vi "all_things_stimulus.vi"(1 "input cluster":T1) -> (0 "output cluster":T2)   [LabVIEW 2010]
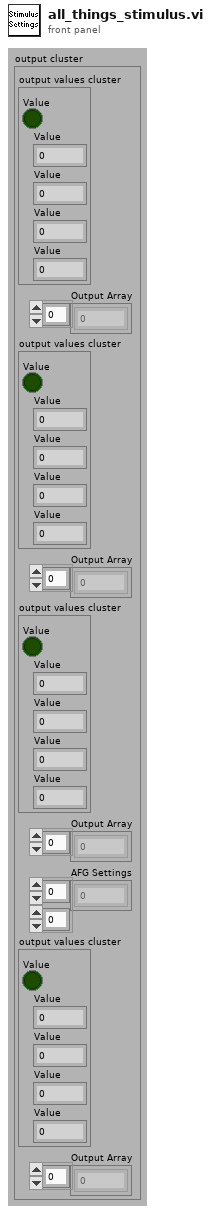
[diagram p1: front panel]
types:
  T1 = cluster{"AFG Settings":dbl[][], "tap timing array":dbl[], "puff timing array":dbl[], "custom timing array":dbl[], "custom 2 timing array":dbl[], cluster{cluster{"Tap":refnum<vi>, "Tap Delay":refnum<vi>, "Tap Interval":refnum<vi>, "Tap Number":refnum<vi>, "Tap Stimulus Method":refnum<vi>}, cluster{"Puff":refnum<vi>, "Puff Delay":refnum<vi>, "Puff Interval":refnum<vi>, "Puff Number":refnum<vi>, "Puff Stimulus Method":refnum<vi>}, cluster{"Custom 1":refnum<vi>, "Custom 1 Delay":refnum<vi>, "Custom 1 Interval":refnum<vi>, "Custom 1 Number":refnum<vi>, "Custom 1 Stimulus Method":refnum<vi>}, cluster{"Custom 2":refnum<vi>, "Custom 2 Delay":refnum<vi>, "Custom 2 Interval":refnum<vi>, "Custom 2 Number":refnum<vi>, "Custom 2 Stimulus Method":refnum<vi>}}, cluster{"Path":refnum<vi>, "Prefix":refnum<vi>, "Type of object to track":refnum<vi>, "Object Contrast (%)":refnum<vi>, "Fill Hysteresis (%)":refnum<vi>, "Maximum Object Size (pixels)":refnum<vi>, "Minimum Object Size (pixels)":refnum<vi>, "Object Size hysteresis (%)":refnum<vi>, "Image Binning":refnum<vi>, "Contour?":refnum<vi>, "Skeletonize?":refnum<vi>, "Frames of Adaptation":refnum<vi>, "Adaptation Rate":refnum<vi>, "Object Border":refnum<vi>, "Image Bit Depth":refnum<vi>, "Bit Depth from Camera?":refnum<vi>, "AFG resource name":refnum<vi>, "IMAQ Camera Interface Name":refnum<vi>, "Device auto-start delay (s)":refnum<vi>, "Number of Image Adaptation Bands":refnum<vi>, "Experiment Duration (s)":refnum<vi>, "Tap":refnum<vi>, "Tap Delay":refnum<vi>, "Tap Interval":refnum<vi>, "Tap Number":refnum<vi>, "Tap Stimulus Method":refnum<vi>, "Advanced Tap Settings":refnum<vi>, "Puff":refnum<vi>, "Puff Delay":refnum<vi>, "Puff Interval":refnum<vi>, "Puff Number":refnum<vi>, "Puff Stimulus Method":refnum<vi>, "Advanced Puff Settings":refnum<vi>, "Custom 1":refnum<vi>, "Custom 1 Delay":refnum<vi>, "Custom 1 Interval":refnum<vi>, "Custom 1 Number":refnum<vi>, "Custom 1 Stimulus Method":refnum<vi>, "Advanced Custom 1 Settings":refnum<vi>, "puff fraction of time between is active":refnum<vi>, "time between puff onset":refnum<vi>, "tap fraction of time between is active":refnum<vi>, "time between tap onset":refnum<vi>, "Tap Train Number":refnum<vi>, "custom 1 fraction of time between is active":refnum<vi>, "time between custom 1 onset":refnum<vi>, "Custom 2":refnum<vi>, "Custom 2 Delay":refnum<vi>, "Custom 2 Interval":refnum<vi>, "Custom 2 Number":refnum<vi>, "Custom 2 Stimulus Method":refnum<vi>, "Advanced Custom 2 Settings":refnum<vi>, "custom 2 fraction of time between is active":refnum<vi>, "time between custom 2 onset":refnum<vi>, "Save":refnum<vi>, "Load":refnum<vi>, "Raw Image Save Interval (s)":refnum<vi>, "Turn on output aggregation?":refnum<vi>, "Turn on Background division algorithm":refnum<vi>, "Turn on external triggering of camera":refnum<vi>}, "output values cluster":cluster{"Value":bool, "Value":dbl, "Value":dbl, "Value":dbl, "Value":u16}, "output values cluster":cluster{"Value":bool, "Value":dbl, "Value":dbl, "Value":dbl, "Value":u16}, "output values cluster":cluster{"Value":bool, "Value":dbl, "Value":dbl, "Value":dbl, "Value":u16}, "output values cluster":cluster{"Value":bool, "Value":dbl, "Value":dbl, "Value":dbl, "Value":u16}}
  T2 = cluster{"output values cluster":cluster{"Value":bool, "Value":dbl, "Value":dbl, "Value":dbl, "Value":u16}, "Output Array":dbl[], "output values cluster":cluster{"Value":bool, "Value":dbl, "Value":dbl, "Value":dbl, "Value":u16}, "Output Array":dbl[], "output values cluster":cluster{"Value":bool, "Value":dbl, "Value":dbl, "Value":dbl, "Value":u16}, "Output Array":dbl[], "AFG Settings":dbl[][], "output values cluster":cluster{"Value":bool, "Value":dbl, "Value":dbl, "Value":dbl, "Value":u16}, "Output Array":dbl[]}
  T3 = cluster{cluster{"Tap":refnum<vi>, "Tap Delay":refnum<vi>, "Tap Interval":refnum<vi>, "Tap Number":refnum<vi>, "Tap Stimulus Method":refnum<vi>}, cluster{"Puff":refnum<vi>, "Puff Delay":refnum<vi>, "Puff Interval":refnum<vi>, "Puff Number":refnum<vi>, "Puff Stimulus Method":refnum<vi>}, cluster{"Custom 1":refnum<vi>, "Custom 1 Delay":refnum<vi>, "Custom 1 Interval":refnum<vi>, "Custom 1 Number":refnum<vi>, "Custom 1 Stimulus Method":refnum<vi>}, cluster{"Custom 2":refnum<vi>, "Custom 2 Delay":refnum<vi>, "Custom 2 Interval":refnum<vi>, "Custom 2 Number":refnum<vi>, "Custom 2 Stimulus Method":refnum<vi>}}
  T4 = cluster{"Path":refnum<vi>, "Prefix":refnum<vi>, "Type of object to track":refnum<vi>, "Object Contrast (%)":refnum<vi>, "Fill Hysteresis (%)":refnum<vi>, "Maximum Object Size (pixels)":refnum<vi>, "Minimum Object Size (pixels)":refnum<vi>, "Object Size hysteresis (%)":refnum<vi>, "Image Binning":refnum<vi>, "Contour?":refnum<vi>, "Skeletonize?":refnum<vi>, "Frames of Adaptation":refnum<vi>, "Adaptation Rate":refnum<vi>, "Object Border":refnum<vi>, "Image Bit Depth":refnum<vi>, "Bit Depth from Camera?":refnum<vi>, "AFG resource name":refnum<vi>, "IMAQ Camera Interface Name":refnum<vi>, "Device auto-start delay (s)":refnum<vi>, "Number of Image Adaptation Bands":refnum<vi>, "Experiment Duration (s)":refnum<vi>, "Tap":refnum<vi>, "Tap Delay":refnum<vi>, "Tap Interval":refnum<vi>, "Tap Number":refnum<vi>, "Tap Stimulus Method":refnum<vi>, "Advanced Tap Settings":refnum<vi>, "Puff":refnum<vi>, "Puff Delay":refnum<vi>, "Puff Interval":refnum<vi>, "Puff Number":refnum<vi>, "Puff Stimulus Method":refnum<vi>, "Advanced Puff Settings":refnum<vi>, "Custom 1":refnum<vi>, "Custom 1 Delay":refnum<vi>, "Custom 1 Interval":refnum<vi>, "Custom 1 Number":refnum<vi>, "Custom 1 Stimulus Method":refnum<vi>, "Advanced Custom 1 Settings":refnum<vi>, "puff fraction of time between is active":refnum<vi>, "time between puff onset":refnum<vi>, "tap fraction of time between is active":refnum<vi>, "time between tap onset":refnum<vi>, "Tap Train Number":refnum<vi>, "custom 1 fraction of time between is active":refnum<vi>, "time between custom 1 onset":refnum<vi>, "Custom 2":refnum<vi>, "Custom 2 Delay":refnum<vi>, "Custom 2 Interval":refnum<vi>, "Custom 2 Number":refnum<vi>, "Custom 2 Stimulus Method":refnum<vi>, "Advanced Custom 2 Settings":refnum<vi>, "custom 2 fraction of time between is active":refnum<vi>, "time between custom 2 onset":refnum<vi>, "Save":refnum<vi>, "Load":refnum<vi>, "Raw Image Save Interval (s)":refnum<vi>, "Turn on output aggregation?":refnum<vi>, "Turn on Background division algorithm":refnum<vi>, "Turn on external triggering of camera":refnum<vi>}
  T5 = cluster{"Value":bool, "Value":dbl, "Value":dbl, "Value":dbl, "Value":u16}
  T6 = cluster{"Tap":refnum<vi>, "Tap Delay":refnum<vi>, "Tap Interval":refnum<vi>, "Tap Number":refnum<vi>, "Tap Stimulus Method":refnum<vi>}
  T7 = cluster{"Puff":refnum<vi>, "Puff Delay":refnum<vi>, "Puff Interval":refnum<vi>, "Puff Number":refnum<vi>, "Puff Stimulus Method":refnum<vi>}
  T8 = cluster{"Custom 1":refnum<vi>, "Custom 1 Delay":refnum<vi>, "Custom 1 Interval":refnum<vi>, "Custom 1 Number":refnum<vi>, "Custom 1 Stimulus Method":refnum<vi>}
  T9 = cluster{"Custom 2":refnum<vi>, "Custom 2 Delay":refnum<vi>, "Custom 2 Interval":refnum<vi>, "Custom 2 Number":refnum<vi>, "Custom 2 Stimulus Method":refnum<vi>}
  T10 = cluster{cluster{"Custom 2":refnum<vi>, "Custom 2 Delay":refnum<vi>, "Custom 2 Interval":refnum<vi>, "Custom 2 Number":refnum<vi>, "Custom 2 Stimulus Method":refnum<vi>}, "output values cluster":cluster{"Value":bool, "Value":dbl, "Value":dbl, "Value":dbl, "Value":u16}, "custom 2 timing array":dbl[], cluster{"Path":refnum<vi>, "Prefix":refnum<vi>, "Type of object to track":refnum<vi>, "Object Contrast (%)":refnum<vi>, "Fill Hysteresis (%)":refnum<vi>, "Maximum Object Size (pixels)":refnum<vi>, "Minimum Object Size (pixels)":refnum<vi>, "Object Size hysteresis (%)":refnum<vi>, "Image Binning":refnum<vi>, "Contour?":refnum<vi>, "Skeletonize?":refnum<vi>, "Frames of Adaptation":refnum<vi>, "Adaptation Rate":refnum<vi>, "Object Border":refnum<vi>, "Image Bit Depth":refnum<vi>, "Bit Depth from Camera?":refnum<vi>, "AFG resource name":refnum<vi>, "IMAQ Camera Interface Name":refnum<vi>, "Device auto-start delay (s)":refnum<vi>, "Number of Image Adaptation Bands":refnum<vi>, "Experiment Duration (s)":refnum<vi>, "Tap":refnum<vi>, "Tap Delay":refnum<vi>, "Tap Interval":refnum<vi>, "Tap Number":refnum<vi>, "Tap Stimulus Method":refnum<vi>, "Advanced Tap Settings":refnum<vi>, "Puff":refnum<vi>, "Puff Delay":refnum<vi>, "Puff Interval":refnum<vi>, "Puff Number":refnum<vi>, "Puff Stimulus Method":refnum<vi>, "Advanced Puff Settings":refnum<vi>, "Custom 1":refnum<vi>, "Custom 1 Delay":refnum<vi>, "Custom 1 Interval":refnum<vi>, "Custom 1 Number":refnum<vi>, "Custom 1 Stimulus Method":refnum<vi>, "Advanced Custom 1 Settings":refnum<vi>, "puff fraction of time between is active":refnum<vi>, "time between puff onset":refnum<vi>, "tap fraction of time between is active":refnum<vi>, "time between tap onset":refnum<vi>, "Tap Train Number":refnum<vi>, "custom 1 fraction of time between is active":refnum<vi>, "time between custom 1 onset":refnum<vi>, "Custom 2":refnum<vi>, "Custom 2 Delay":refnum<vi>, "Custom 2 Interval":refnum<vi>, "Custom 2 Number":refnum<vi>, "Custom 2 Stimulus Method":refnum<vi>, "Advanced Custom 2 Settings":refnum<vi>, "custom 2 fraction of time between is active":refnum<vi>, "time between custom 2 onset":refnum<vi>, "Save":refnum<vi>, "Load":refnum<vi>, "Raw Image Save Interval (s)":refnum<vi>, "Turn on output aggregation?":refnum<vi>, "Turn on Background division algorithm":refnum<vi>, "Turn on external triggering of camera":refnum<vi>}}
  T11 = cluster{cluster{"Puff":refnum<vi>, "Puff Delay":refnum<vi>, "Puff Interval":refnum<vi>, "Puff Number":refnum<vi>, "Puff Stimulus Method":refnum<vi>}, "output values cluster":cluster{"Value":bool, "Value":dbl, "Value":dbl, "Value":dbl, "Value":u16}, "puff timing array":dbl[], cluster{"Path":refnum<vi>, "Prefix":refnum<vi>, "Type of object to track":refnum<vi>, "Object Contrast (%)":refnum<vi>, "Fill Hysteresis (%)":refnum<vi>, "Maximum Object Size (pixels)":refnum<vi>, "Minimum Object Size (pixels)":refnum<vi>, "Object Size hysteresis (%)":refnum<vi>, "Image Binning":refnum<vi>, "Contour?":refnum<vi>, "Skeletonize?":refnum<vi>, "Frames of Adaptation":refnum<vi>, "Adaptation Rate":refnum<vi>, "Object Border":refnum<vi>, "Image Bit Depth":refnum<vi>, "Bit Depth from Camera?":refnum<vi>, "AFG resource name":refnum<vi>, "IMAQ Camera Interface Name":refnum<vi>, "Device auto-start delay (s)":refnum<vi>, "Number of Image Adaptation Bands":refnum<vi>, "Experiment Duration (s)":refnum<vi>, "Tap":refnum<vi>, "Tap Delay":refnum<vi>, "Tap Interval":refnum<vi>, "Tap Number":refnum<vi>, "Tap Stimulus Method":refnum<vi>, "Advanced Tap Settings":refnum<vi>, "Puff":refnum<vi>, "Puff Delay":refnum<vi>, "Puff Interval":refnum<vi>, "Puff Number":refnum<vi>, "Puff Stimulus Method":refnum<vi>, "Advanced Puff Settings":refnum<vi>, "Custom 1":refnum<vi>, "Custom 1 Delay":refnum<vi>, "Custom 1 Interval":refnum<vi>, "Custom 1 Number":refnum<vi>, "Custom 1 Stimulus Method":refnum<vi>, "Advanced Custom 1 Settings":refnum<vi>, "puff fraction of time between is active":refnum<vi>, "time between puff onset":refnum<vi>, "tap fraction of time between is active":refnum<vi>, "time between tap onset":refnum<vi>, "Tap Train Number":refnum<vi>, "custom 1 fraction of time between is active":refnum<vi>, "time between custom 1 onset":refnum<vi>, "Custom 2":refnum<vi>, "Custom 2 Delay":refnum<vi>, "Custom 2 Interval":refnum<vi>, "Custom 2 Number":refnum<vi>, "Custom 2 Stimulus Method":refnum<vi>, "Advanced Custom 2 Settings":refnum<vi>, "custom 2 fraction of time between is active":refnum<vi>, "time between custom 2 onset":refnum<vi>, "Save":refnum<vi>, "Load":refnum<vi>, "Raw Image Save Interval (s)":refnum<vi>, "Turn on output aggregation?":refnum<vi>, "Turn on Background division algorithm":refnum<vi>, "Turn on external triggering of camera":refnum<vi>}}
  T12 = cluster{cluster{"Custom 1":refnum<vi>, "Custom 1 Delay":refnum<vi>, "Custom 1 Interval":refnum<vi>, "Custom 1 Number":refnum<vi>, "Custom 1 Stimulus Method":refnum<vi>}, "output values cluster":cluster{"Value":bool, "Value":dbl, "Value":dbl, "Value":dbl, "Value":u16}, "custom timing array":dbl[], cluster{"Path":refnum<vi>, "Prefix":refnum<vi>, "Type of object to track":refnum<vi>, "Object Contrast (%)":refnum<vi>, "Fill Hysteresis (%)":refnum<vi>, "Maximum Object Size (pixels)":refnum<vi>, "Minimum Object Size (pixels)":refnum<vi>, "Object Size hysteresis (%)":refnum<vi>, "Image Binning":refnum<vi>, "Contour?":refnum<vi>, "Skeletonize?":refnum<vi>, "Frames of Adaptation":refnum<vi>, "Adaptation Rate":refnum<vi>, "Object Border":refnum<vi>, "Image Bit Depth":refnum<vi>, "Bit Depth from Camera?":refnum<vi>, "AFG resource name":refnum<vi>, "IMAQ Camera Interface Name":refnum<vi>, "Device auto-start delay (s)":refnum<vi>, "Number of Image Adaptation Bands":refnum<vi>, "Experiment Duration (s)":refnum<vi>, "Tap":refnum<vi>, "Tap Delay":refnum<vi>, "Tap Interval":refnum<vi>, "Tap Number":refnum<vi>, "Tap Stimulus Method":refnum<vi>, "Advanced Tap Settings":refnum<vi>, "Puff":refnum<vi>, "Puff Delay":refnum<vi>, "Puff Interval":refnum<vi>, "Puff Number":refnum<vi>, "Puff Stimulus Method":refnum<vi>, "Advanced Puff Settings":refnum<vi>, "Custom 1":refnum<vi>, "Custom 1 Delay":refnum<vi>, "Custom 1 Interval":refnum<vi>, "Custom 1 Number":refnum<vi>, "Custom 1 Stimulus Method":refnum<vi>, "Advanced Custom 1 Settings":refnum<vi>, "puff fraction of time between is active":refnum<vi>, "time between puff onset":refnum<vi>, "tap fraction of time between is active":refnum<vi>, "time between tap onset":refnum<vi>, "Tap Train Number":refnum<vi>, "custom 1 fraction of time between is active":refnum<vi>, "time between custom 1 onset":refnum<vi>, "Custom 2":refnum<vi>, "Custom 2 Delay":refnum<vi>, "Custom 2 Interval":refnum<vi>, "Custom 2 Number":refnum<vi>, "Custom 2 Stimulus Method":refnum<vi>, "Advanced Custom 2 Settings":refnum<vi>, "custom 2 fraction of time between is active":refnum<vi>, "time between custom 2 onset":refnum<vi>, "Save":refnum<vi>, "Load":refnum<vi>, "Raw Image Save Interval (s)":refnum<vi>, "Turn on output aggregation?":refnum<vi>, "Turn on Background division algorithm":refnum<vi>, "Turn on external triggering of camera":refnum<vi>}, "AFG Settings":dbl[][]}
  T13 = cluster{cluster{"Tap":refnum<vi>, "Tap Delay":refnum<vi>, "Tap Interval":refnum<vi>, "Tap Number":refnum<vi>, "Tap Stimulus Method":refnum<vi>}, "output values cluster":cluster{"Value":bool, "Value":dbl, "Value":dbl, "Value":dbl, "Value":u16}, "tap timing array":dbl[], cluster{"Path":refnum<vi>, "Prefix":refnum<vi>, "Type of object to track":refnum<vi>, "Object Contrast (%)":refnum<vi>, "Fill Hysteresis (%)":refnum<vi>, "Maximum Object Size (pixels)":refnum<vi>, "Minimum Object Size (pixels)":refnum<vi>, "Object Size hysteresis (%)":refnum<vi>, "Image Binning":refnum<vi>, "Contour?":refnum<vi>, "Skeletonize?":refnum<vi>, "Frames of Adaptation":refnum<vi>, "Adaptation Rate":refnum<vi>, "Object Border":refnum<vi>, "Image Bit Depth":refnum<vi>, "Bit Depth from Camera?":refnum<vi>, "AFG resource name":refnum<vi>, "IMAQ Camera Interface Name":refnum<vi>, "Device auto-start delay (s)":refnum<vi>, "Number of Image Adaptation Bands":refnum<vi>, "Experiment Duration (s)":refnum<vi>, "Tap":refnum<vi>, "Tap Delay":refnum<vi>, "Tap Interval":refnum<vi>, "Tap Number":refnum<vi>, "Tap Stimulus Method":refnum<vi>, "Advanced Tap Settings":refnum<vi>, "Puff":refnum<vi>, "Puff Delay":refnum<vi>, "Puff Interval":refnum<vi>, "Puff Number":refnum<vi>, "Puff Stimulus Method":refnum<vi>, "Advanced Puff Settings":refnum<vi>, "Custom 1":refnum<vi>, "Custom 1 Delay":refnum<vi>, "Custom 1 Interval":refnum<vi>, "Custom 1 Number":refnum<vi>, "Custom 1 Stimulus Method":refnum<vi>, "Advanced Custom 1 Settings":refnum<vi>, "puff fraction of time between is active":refnum<vi>, "time between puff onset":refnum<vi>, "tap fraction of time between is active":refnum<vi>, "time between tap onset":refnum<vi>, "Tap Train Number":refnum<vi>, "custom 1 fraction of time between is active":refnum<vi>, "time between custom 1 onset":refnum<vi>, "Custom 2":refnum<vi>, "Custom 2 Delay":refnum<vi>, "Custom 2 Interval":refnum<vi>, "Custom 2 Number":refnum<vi>, "Custom 2 Stimulus Method":refnum<vi>, "Advanced Custom 2 Settings":refnum<vi>, "custom 2 fraction of time between is active":refnum<vi>, "time between custom 2 onset":refnum<vi>, "Save":refnum<vi>, "Load":refnum<vi>, "Raw Image Save Interval (s)":refnum<vi>, "Turn on output aggregation?":refnum<vi>, "Turn on Background division algorithm":refnum<vi>, "Turn on external triggering of camera":refnum<vi>}}
  T14 = cluster{"output values cluster":cluster{"Value":bool, "Value":dbl, "Value":dbl, "Value":dbl, "Value":u16}, "Output Array":dbl[]}
  T15 = cluster{"output values cluster":cluster{"Value":bool, "Value":dbl, "Value":dbl, "Value":dbl, "Value":u16}, "Output Array":dbl[], "AFG Settings":dbl[][]}
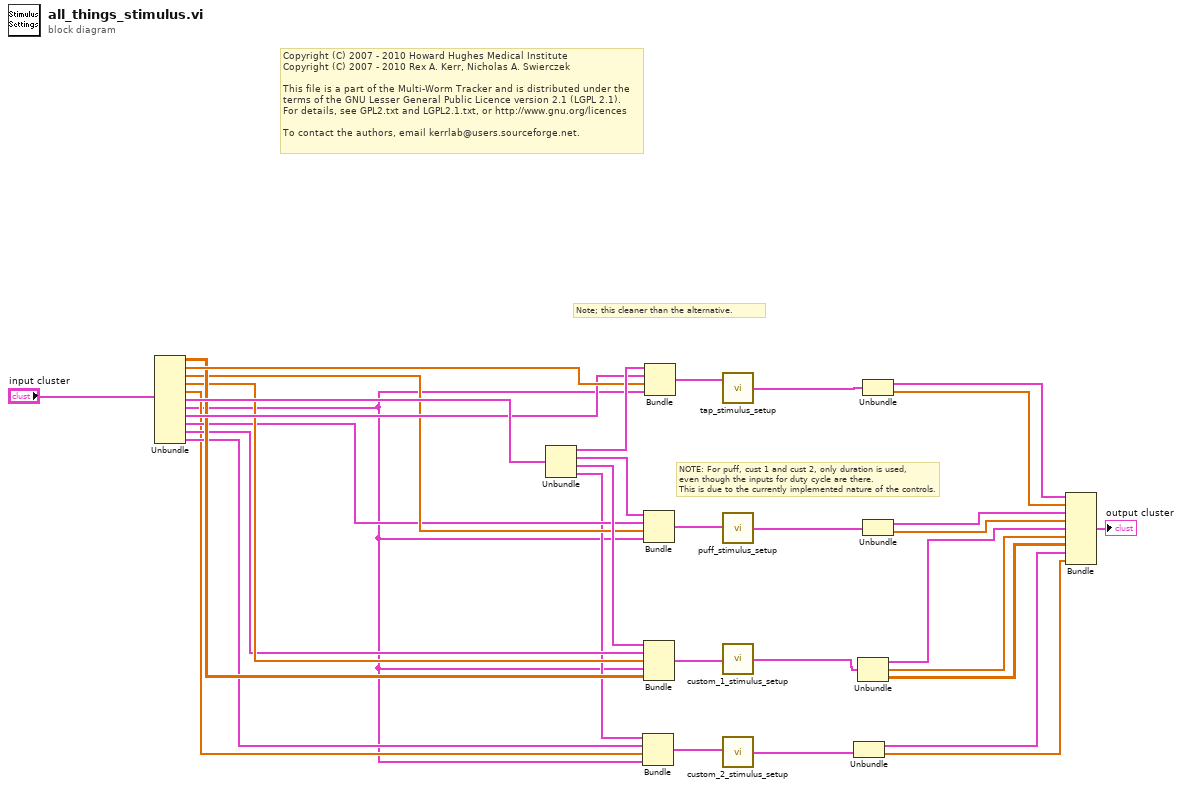
[diagram p0: block diagram]
diagram:
  # "Copyright (C) 2007 - 2010 Howard Hughes Medical Institute\nCopyright (C) 2007 - 2010 Rex A. Kerr, Nicholas A. Swierczek\n \nThis file is a part of the Multi-Worm Tracker and is distributed under the\nterms of the GNU Lesser General Public Licence version 2.1 (LGPL 2.1).\nFor details, see GPL2.txt and LGPL2.1.txt, or http://www.gnu.org/licences\n \nTo contact the authors, email kerrlab@users.sourceforge.net."
  # "NOTE: For puff, cust 1 and cust 2, only duration is used,\neven though the inputs for duty cycle are there.\nThis is due to the currently implemented nature of the controls."
  # "Note; this cleaner than the alternative."
  n1 = Unbundle("input cluster") -> ("AFG Settings"=w15:dbl[][], "tap timing array"=w18:dbl[], "puff timing array"=w14:dbl[], "custom timing array"=w13:dbl[], "custom 2 timing array"=w8:dbl[], w17:T3, w7:T4, "output values cluster"=w16:T5, "output values cluster"=w12:T5, "output values cluster"=w11:T5, "output values cluster"=w9:T5)
  n2 = Unbundle(w17) -> (w34:T6, w33:T7, w31:T8, w10:T9)
  n3 = Bundle(w10, "output values cluster"=w9, "custom 2 timing array"=w8, w7) -> (w6:T10)  [unwired: 1 in]
  n4 = Bundle(w33, "output values cluster"=w12, "puff timing array"=w14, w7) -> (w32:T11)  [unwired: 1 in]
  n5 = Bundle(w31, "output values cluster"=w11, "custom timing array"=w13, w7, "AFG Settings"=w15) -> (w29:T12)  [unwired: 1 in]
  n6 = Bundle(w34, "output values cluster"=w16, "tap timing array"=w18, w7) -> (w30:T13)  [unwired: 1 in]
  n7 = call "tap_stimulus_setup.vi"("input cluster"=w30) -> ("output cluster"=w26:T14)
  n8 = call "puff_stimulus_setup.vi"("input cluster"=w32) -> ("output cluster"=w27:T14)
  n9 = call "custom_1_stimulus_setup.vi"("input cluster"=w29) -> ("output cluster"=w28:T15)
  n10 = call "custom_2_stimulus_setup.vi"("input cluster"=w6) -> ("output cluster"=w5:T14)
  n11 = Unbundle(w5) -> ("output values cluster"=w4:T5, "Output Array"=w3:dbl[])
  n12 = Unbundle(w28) -> ("output values cluster"=w21:T5, "Output Array"=w20:dbl[], "AFG Settings"=w19:dbl[][])
  n13 = Unbundle(w26) -> ("output values cluster"=w25:T5, "Output Array"=w24:dbl[])
  n14 = Unbundle(w27) -> ("output values cluster"=w23:T5, "Output Array"=w22:dbl[])
  n15 = Bundle("output values cluster"=w25, "Output Array"=w24, "output values cluster"=w23, "Output Array"=w22, "output values cluster"=w21, "Output Array"=w20, "AFG Settings"=w19, "output values cluster"=w4, "Output Array"=w3) -> (→"output cluster":T2)  [unwired: 1 in]
